vi "set_motion_fault_by_name.vi"(8 "error in (no error)":errorcluster caption="错误输入（无错误）", 9 "fault?":bool, 10 "name":string, 11 "MotorSystem输入":refnum<class "MotorSystem.lvclass">) -> (0 "error out":errorcluster caption="错误输出", 3 "MotorSystem输出":refnum<class "MotorSystem.lvclass">)   [LabVIEW 2016, in "MotionControl.lvlib" / "MotorSystem.lvclass"]
uses:
  <userlib>/MotionControl/MotorSystem/MotorSystem.lvclass
  <userlib>/MotionControl/MotorSystem/MotorSystem.lvclass/MotorSystem.ctl
  <userlib>/MotionControl/OneMotion/OneMotion.lvclass/OneMotion.ctl
  <userlib>/MotionControl/OneMotion/OneMotion.lvclass
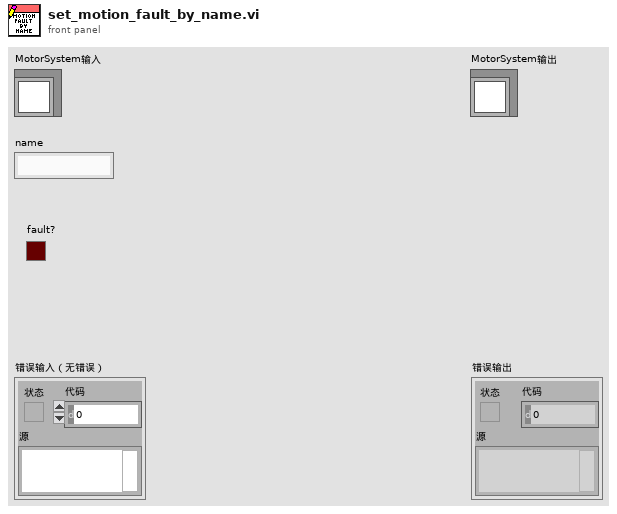
[diagram p1: front panel]
types:
  T1 = typedef "MotionControl.lvlib/MotorSystem.lvclass/MotionCluster.ctl" = cluster{"OneMotion.lvclass":refnum<class "OneMotion.lvclass">, "connected?":bool, "default enabled?":bool, "enabled?":bool}
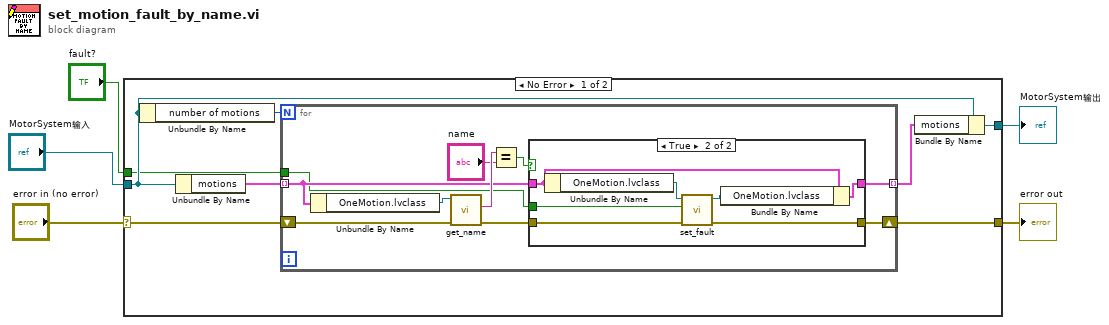
[diagram p0: block diagram]
diagram:
  n1 = case shown="No Error" "error in (no error)" {
    selector: "error in (no error)" -> [w7 w33]
    tunnel: [w6 w33] -> w4
    tunnel: [w13 w34] -> w2
    tunnel: "MotorSystem输入" -> [w12 w34]
    tunnel: "fault?" -> [w8 _]
    frame No Error {
      n2 = Unbundle By Name(w12) -> ("number of motions"=w11:i32)
      n3 = Unbundle By Name(w12) -> ("motions"=w10:T1[])
      n4 = for {
        N: w11 -> [_]
        tunnel: w10 -> [w19] mode=indexing
        tunnel: [w18] -> w9 mode=indexing
        tunnel: w8 -> [w17]
        shift-right: [w14] -> w6
        shift-left: w7 -> [w16]
        n5 = Unbundle By Name(w19) -> ("OneMotion.lvclass"=w23:refnum<class "OneMotion.lvclass">)
        n6 = call-dynamic "get_name.vi"("error in (no error)"=w16, "OneMotion输入"=w23) -> ("error out"=w15:errorcluster, "name"=w22:string)  [unwired: 7 in, 1 out]
        n7 = Equal?(x=w22, y="name") -> (x = y?=w20:bool)
        n8 = case shown="True" w20 {
          tunnel: w19 -> [w25 w30]
          tunnel: [w25 w28] -> w18
          tunnel: w17 -> [_ w31]
          tunnel: w15 -> [w24 w27]
          tunnel: [w24 w26] -> w14
          frame False {
          }
          frame True {
            n9 = Unbundle By Name(w30) -> ("OneMotion.lvclass"=w32:refnum<class "OneMotion.lvclass">)
            n10 = call <userlib>:"set_fault.vi"("error in (no error)"=w27, "fault?"=w31, "OneMotion输入"=w32) -> ("error out"=w26:errorcluster, "OneMotion输出"=w29:refnum<class "OneMotion.lvclass">)  [unwired: 7 in]
            n11 = Bundle By Name(cluster=w30, "OneMotion.lvclass"=w29) -> (w28:T1)
          }
        }
      }
      n12 = Bundle By Name(cluster=w12, "motions"=w9) -> (w13:refnum<class "MotorSystem.lvclass">)
    }
    frame Error {
    }
  }
  "error out" <- w4
  "MotorSystem输出" <- w2
